vi "Load Vorbis.vi"(8 "error in (no error)":errorcluster, 11 "Path":path) -> (0 "error out":errorcluster, 1 "data":waveform(i16)[](array[waveform]), 2 "Sample Rate (Hz)":u32, 3 "Channels":u32, 5 "Length (Samples)":u64)   [LabVIEW 2019, in "LabVIEW Audio Codecs.lvlib"]
doc: "Loads an Ogg Vorbis file from disk.\n\n<b>Priority:</b> Background priority (lowest)"
uses:
  LabVIEW Audio Codecs.lvlib
  labview_audio_codecs_x86.dll
  labview_audio_codecs_x64.dll
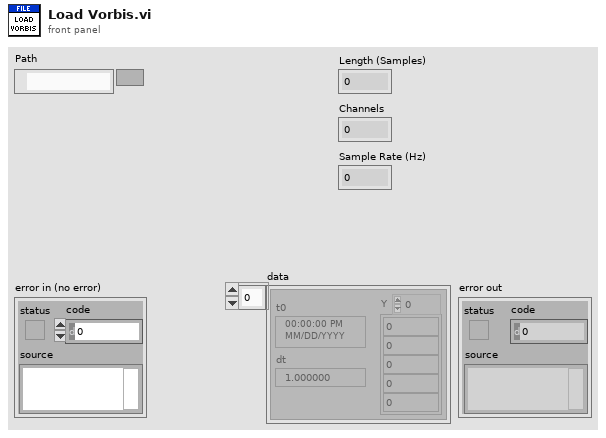
[diagram p1: front panel]
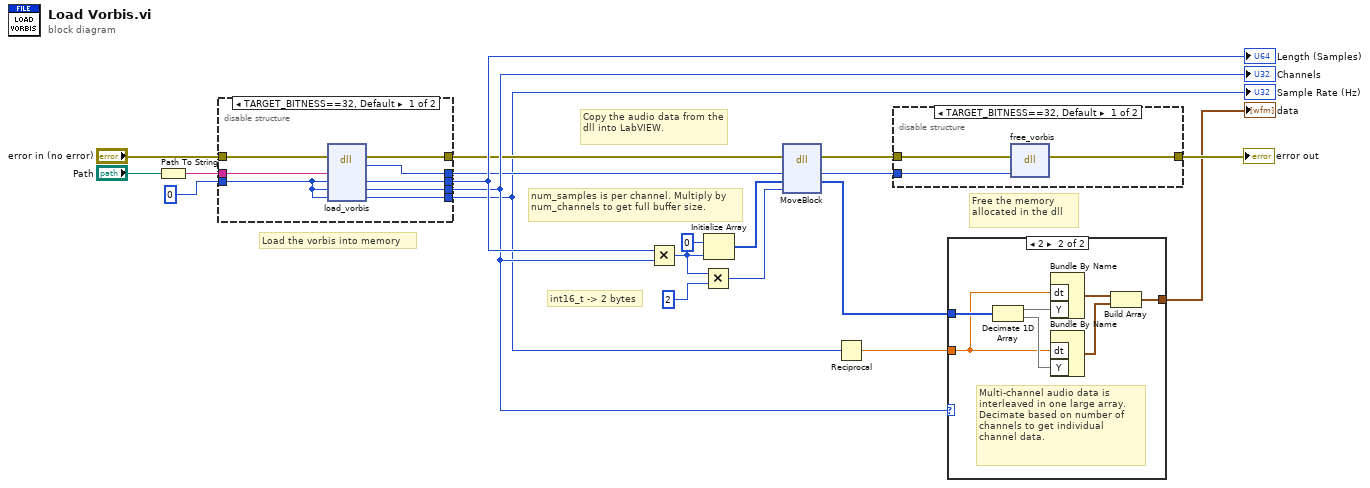
[diagram p0: block diagram]
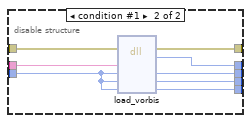
[diagram p2: hidden frame]
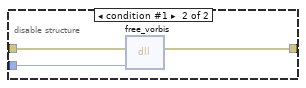
[diagram p3: hidden frame]
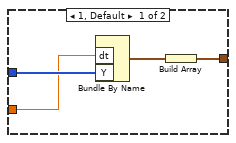
[diagram p4: hidden frame]
diagram:
  # "num_samples is per channel. Multiply by num_channels to get full buffer size."
  # "Free the memory allocated in the dll"
  # "Copy the audio data from the dll into LabVIEW."
  # "Load the vorbis into memory"
  # "int16_t -> 2 bytes"
  n1 = Path To String(path="Path") -> (string=w14:string)
  n2 = disable-structure shown="TARGET_BITNESS==32, Default" {
    disable-tunnel: "error in (no error)" -> [w28 w36]
    disable-tunnel: [w26 w34] -> w17
    disable-tunnel: [w25 w33] -> w16
    disable-tunnel: [w24 w32] -> w2
    disable-tunnel: w14 -> [w22 w30]
    disable-tunnel: [w23 w31] -> w12
    disable-tunnel: [w27 w35] -> w10
    disable-tunnel: 0 ("num_samples") -> [w21 w29]
    frame condition #0 (active) {
      n3 = dll-call lib="C:/github/dataflowg/labview-simcity-2000-toolkit/src/Sound/LabVIEW Audio Codecs/labview_audio_codecs_x86.*" fn="load_vorbis"(error in=w28, "file_name"=w22, "num_samples"=w21, "channels"=w21, "sample_rate"=w21) -> (error out=w27:errorcluster, "return type"=w23:i64, "num_samples"=w26:i32, "channels"=w25:i32, "sample_rate"=w24:i32)  [unwired: 3 in, 1 out]
    }
    frame condition #1 {
      n4 = dll-call lib="C:/github/dataflowg/labview-audio-codecs/src/LabVIEW/LabVIEW Audio Codecs/labview_audio_codecs_x64.*" fn="load_vorbis"(error in=w36, "file_name"=w30, "num_samples"=w29, "channels"=w29, "sample_rate"=w29) -> (error out=w35:errorcluster, "return type"=w31:i64, "num_samples"=w34:i32, "channels"=w33:i32, "sample_rate"=w32:i32)  [unwired: 3 in, 1 out]
    }
  }
  "Length (Samples)" <- w17
  "Channels" <- w16
  "Sample Rate (Hz)" <- w2
  n5 = Multiply(x=w17, y=w16) -> (x*y=w3:i32)
  n6 = Multiply(x=w3, y=u64 2) -> (x*y=w8:u64)
  n7 = Initialize Array(i16 0 ("num_samples"), w3) -> (w11:i16[])
  n8 = dll-call lib="LabVIEW" fn="MoveBlock"(error in=w10, "Address (Pointer)"=w12, "Destination"=w11, "Size"=w8) -> (error out=w6:errorcluster, "Address (Pointer)"=w7:i64, "Destination"=w5:i16[])  [unwired: 4 in, 1 out]
  n9 = Reciprocal(x=w2) -> (1/x=w1:dbl)
  n10 = disable-structure shown="TARGET_BITNESS==32, Default" {
    disable-tunnel: [w39 w42] -> w19
    disable-tunnel: w7 -> [w38 w41]
    disable-tunnel: w6 -> [w37 w40]
    frame condition #0 (active) {
      n11 = dll-call lib="C:/github/dataflowg/labview-simcity-2000-toolkit/src/Sound/LabVIEW Audio Codecs/labview_audio_codecs_x86.*" fn="free_vorbis"(error in=w37, "Address (Pointer)"=w38) -> (error out=w39:errorcluster)  [unwired: 4 in, 1 out]
    }
    frame condition #1 {
      n12 = dll-call lib="C:/github/dataflowg/labview-audio-codecs/src/LabVIEW/LabVIEW Audio Codecs/labview_audio_codecs_x64.*" fn="free_vorbis"(error in=w40, "Address (Pointer)"=w41) -> (error out=w42:errorcluster)  [unwired: 4 in, 1 out]
    }
  }
  "error out" <- w19
  n13 = case shown="2" w16 {
    tunnel: w5 -> [w46 w53]
    tunnel: [w45 w48] -> w15
    tunnel: w1 -> [w43 w47]
    frame 1, Default {
      n14 = Bundle By Name("dt"=w43, "Y"=w46) -> (w44:waveform(i16))  [unwired: 1 in]
      n15 = Build Array(w44) -> (w45:waveform(i16)[])
    }
    frame 2 {
      # "Multi-channel audio data is interleaved in one large array. Decimate based on number of channels to get individual channel data."
      n16 = Decimate 1D Array(w53) -> (w52:i16[], w51:i16[])
      n17 = Bundle By Name("dt"=w47, "Y"=w52) -> (w50:waveform(i16))  [unwired: 1 in]
      n18 = Bundle By Name("dt"=w47, "Y"=w51) -> (w49:waveform(i16))  [unwired: 1 in]
      n19 = Build Array(w50, w49) -> (w48:waveform(i16)[])
    }
  }
  "data" <- w15
